vi "LoadReferenceMonitorData.vi"(8 "错误输入（无错误）":errorcluster, 9 "MPM":refnum<k24>[](array[refnum]), 10 "TSL":refnum<k24>, 11 "SPU":refnum<k24>) -> (0 "错误输出":errorcluster, 2 "monitor":sgl[](array[numeric]), 3 "trigger":sgl[](array[numeric]))   [LabVIEW 2017]
uses:
  D:/test/PDLSTS/LV_PDL LvVer17.0/LV_PDL_x64/DLL/InstrumentDLL.dll
  DLL/InstrumentDLL.dll
  Share/MPM_PowerMonitorType.vi
  Share/Actual_step.vi
panel:
  out "size(s) 2":i32
  out "size(s)":i32
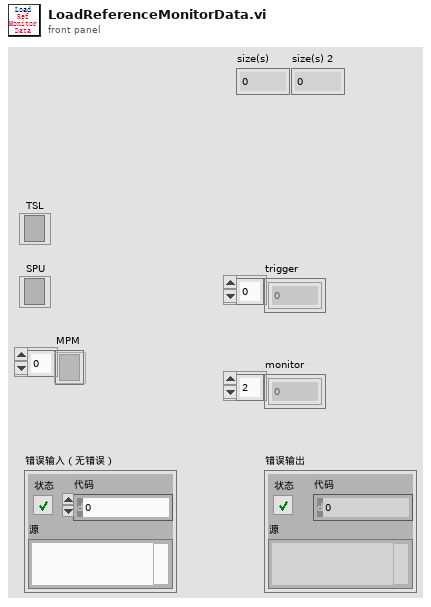
[diagram p1: front panel]
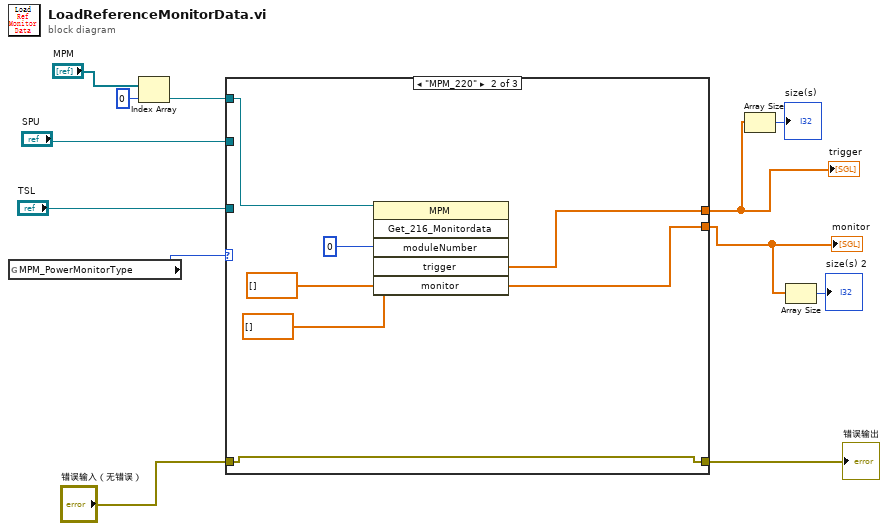
[diagram p0: block diagram]
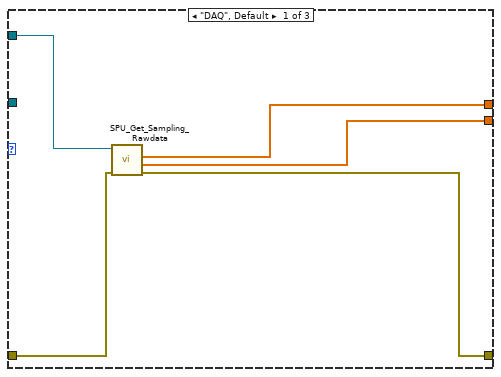
[diagram p2: hidden frame]
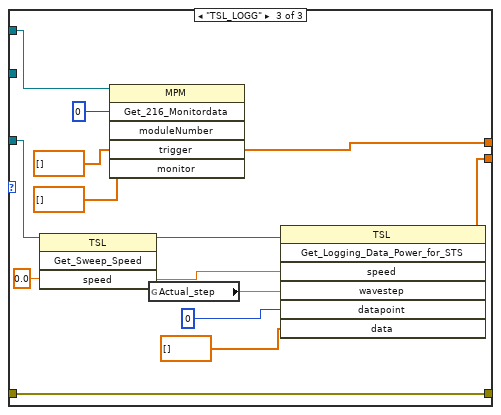
[diagram p3: hidden frame]
diagram:
  n1 = global read "MPM_PowerMonitorType.vi" "MPM_PowerMonitorType"() -> (w12:enum16{"DAQ", "MPM_220", "TSL_LOGG"})
  n2 = Index Array(array="MPM", index=0 ("索引")) -> (element=w6:refnum<k24>)
  n3 = case shown="\"MPM_220\"" w12 {
    tunnel: "错误输入（无错误）" -> [w17 w23 w37]
    tunnel: "SPU" -> [w16 _ _]
    tunnel: [w15 w19 w34] -> w4
    tunnel: [w14 w18 w27] -> w2
    tunnel: [w13 w23 w37] -> w9
    tunnel: w6 -> [_ w24 w38]
    tunnel: "TSL" -> [_ _ w30]
    frame "DAQ", Default {
      n4 = call "SPU_Get_Sampling_Rawdata.vi"("错误输入（无错误）"=w17, "SPU"=w16) -> ("error out"=w13:errorcluster, "monitor"=w14:sgl[], "trigger"=w15:sgl[])  [unwired: 5 in, 1 out]
    }
    frame "MPM_220" {
      n5 = invoke class="MPM" method="Get_216_Monitordata"(reference=w24, "moduleNumber"=0, "trigger"=sgl[] [], "monitor"=sgl[] []) -> ("trigger"=w19:sgl[], "monitor"=w18:sgl[])  [unwired: 2 in, 4 out]
    }
    frame "TSL_LOGG" {
      n6 = invoke class="TSL" method="Get_Sweep_Speed"(reference=w30, "speed"=0.0) -> (reference out=w26:refnum<k24>, "speed"=w29:dbl)  [unwired: 2 in, 2 out]
      n7 = invoke class="MPM" method="Get_216_Monitordata"(reference=w38, "moduleNumber"=0, "trigger"=sgl[] [], "monitor"=sgl[] []) -> ("trigger"=w34:sgl[])  [unwired: 2 in, 5 out]
      n8 = global read "Actual_step.vi" "Actual_step"() -> (w25:dbl)
      n9 = invoke class="TSL" method="Get_Logging_Data_Power_for_STS"(reference=w26, "speed"=w29, "wavestep"=w25, "datapoint"=0, "data"=sgl[] []) -> ("data"=w27:sgl[])  [unwired: 2 in, 6 out]
    }
  }
  "错误输出" <- w9
  "trigger" <- w4
  "monitor" <- w2
  n10 = Array Size(array=w4) -> (size(s)=→"size(s)":i32)
  n11 = Array Size(array=w2) -> (size(s)=→"size(s) 2":i32)
